vi "DeCoF wait for prompt TCP-socket.vi"(6 "error in (no error)":errorcluster, 7 "time out (ms)":i32=1000, 9 "Connection ID":refnum<k5>) -> (0 "error out":errorcluster, 1 "timed out?":bool, 2 "answer string":string, 3 "Connection ID out":refnum<k5>, 4 "complete answer":string)   [LabVIEW 2013]
doc: "This VI collects the input from the TCP/IP connection until the prompt string is found or the timeout expires.\nThe answer string contains the complete collected string minus the prompt, if found."
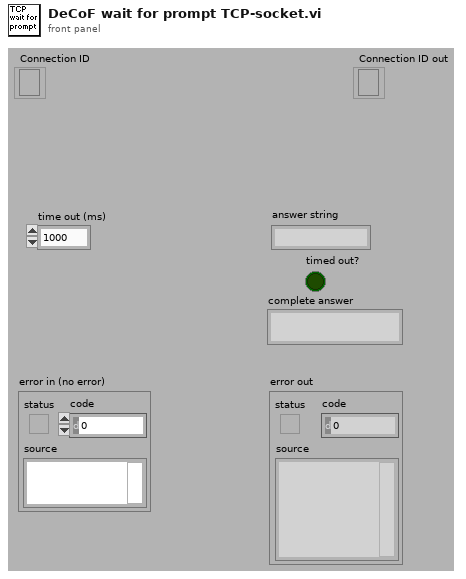
[diagram p1: front panel]
types:
  T1 = enum16{"Standard", "Buffered", "CRLF", "Immediate"}
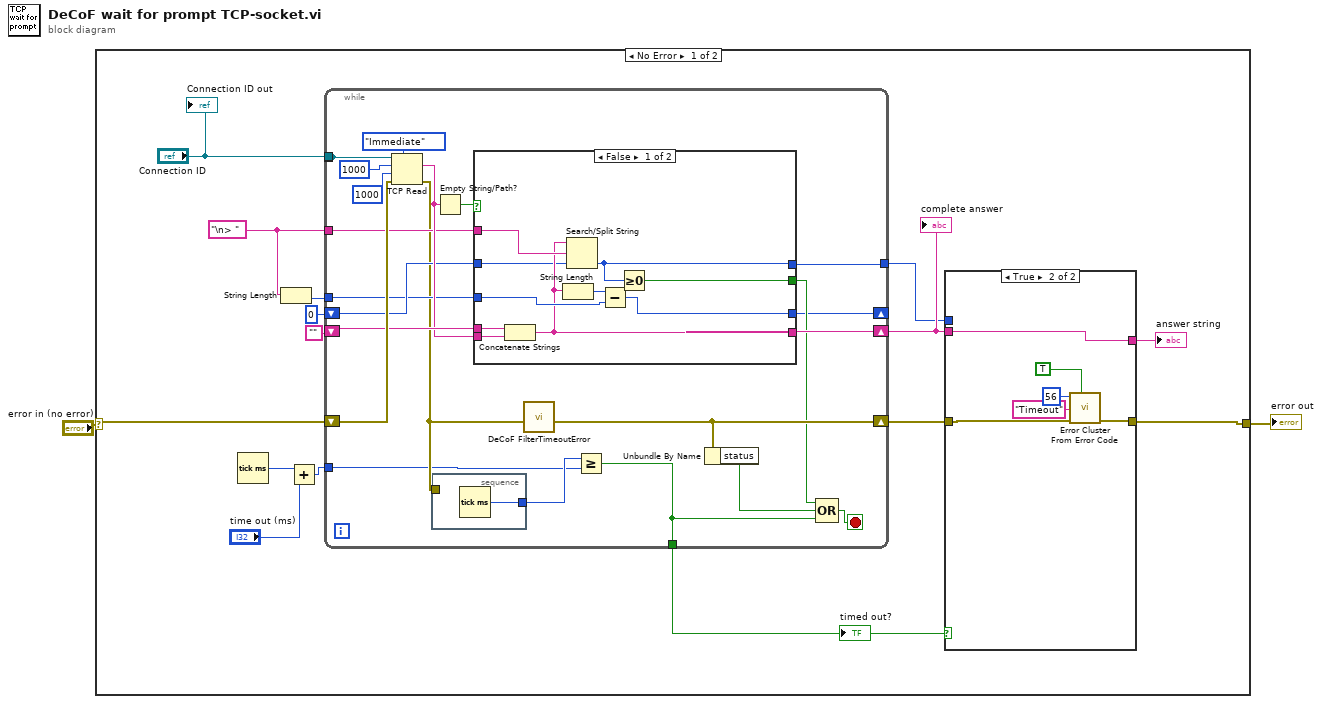
[diagram p0: block diagram]
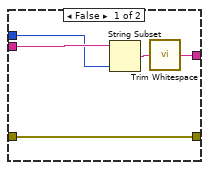
[diagram p2: hidden frame]
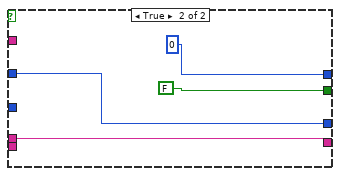
[diagram p3: hidden frame]
diagram:
  n1 = case shown="No Error" "error in (no error)" {
    selector: "error in (no error)" -> [w16 w66]
    tunnel: [w12 w66] -> w1
    frame No Error {
      w9 = "\n> " ("prompt")
      n2 = Tick Count (ms)() -> (millisecond timer value=w7:u32)
      n3 = String Length(string=w9) -> (length=w8:i32)
      n4 = Add(x=w7, y="time out (ms)") -> (x+y=w5:u32)
      n5 = while {
        shift-right: [w41] -> w11
        shift-left: w16 -> [w47]
        tunnel: [w29] -> _
        shift-right: [w35] -> _
        shift-left: 0 -> [w38]
        tunnel: w9 -> [w39]
        shift-right: [w45] -> w14
        shift-left: "" -> [w44]
        tunnel: [w36] -> w10
        tunnel: w8 -> [w34]
        tunnel: w5 -> [w31]
        tunnel: [w30] -> w4
        tunnel: "Connection ID" -> [w29]
        stop <- w50 stop-if-true
        n6 = TCP Read(connection ID=w29, bytes to read=1000, error in (no error)=w47, 7:T1."Immediate" ("mode (standard)"), 9:1000 ("timeout ms (25000)")) -> (data out=w42:string, error out=w33:errorcluster)  [unwired: 1 out]
        n7 = stacked-sequence {
          tunnel: w33 -> [_]
          tunnel: [w51] -> w32
          frame #0 {
            n8 = Tick Count (ms)() -> (millisecond timer value=w51:u32)
          }
        }
        n9 = Empty String/Path?(string/path=w42) -> (empty?=w40:bool)
        n10 = case shown="False" w40 {
          tunnel: [w55 w65] -> w45
          tunnel: w44 -> [w59 w65]
          tunnel: w42 -> [w61 _]
          tunnel: w39 -> [w60 _]
          tunnel: w38 -> [w52 w64]
          tunnel: [w53 FALSE] -> w37
          tunnel: [w54 0 ("offset of match")] -> w36
          tunnel: [w56 w64] -> w35
          tunnel: w34 -> [w57 _]
          frame False {
            n11 = Concatenate Strings(w59, w61) -> (w55:string)
            n12 = String Length(string=w55) -> (length=w58:i32)
            n13 = Search/Split String(string=w55, search string/char (-)=w60, offset (0)=w52) -> (offset of match=w54:i32)  [unwired: 2 out]
            n14 = Subtract(x=w58, y=w57) -> (x-y=w56:i32)
            n15 = Greater Or Equal To 0?(x=w54) -> (x >= 0?=w53:bool)
          }
          frame True {
          }
        }
        n16 = call "DeCoF FilterTimeoutError.vi"("error in (no error)"=w33) -> ("error out"=w41:errorcluster)  [unwired: 5 in, 1 out]
        n17 = Greater Or Equal?(x=w32, y=w31) -> (x >= y?=w30:bool)
        n18 = Unbundle By Name(w41) -> ("status"=w43:bool)
        n19 = Compound Arithmetic op=OR(w37, w43, w30) -> (w50:bool)
      }
      "complete answer" <- w14
      "timed out?" <- w4
      n20 = case shown="True" w4 {
        tunnel: w14 -> [w22 w28]
        tunnel: [w20 w28] -> w13
        tunnel: [w19 w26] -> w12
        tunnel: w11 -> [w19 w27]
        tunnel: w10 -> [w18 _]
        frame False {
          n21 = String Subset(string=w22, length (rest)=w18) -> (substring=w21:string)  [unwired: 1 in]
          n22 = call <vilib>:"Trim Whitespace.vi"("string"=w21) -> ("trimmed string"=w20:string)  [unwired: 1 in]
        }
        frame True {
          n23 = call <vilib>:"Error Cluster From Error Code.vi"("show call chain? (False)"=TRUE, "error in (no error)"=w27, "error message (\"\")"="Timeout" ("error message (\"\")"), "error code (0)"=56) -> ("error out"=w26:errorcluster)  [unwired: 5 in]
        }
      }
      "answer string" <- w13
      "Connection ID out" <- "Connection ID"
    }
    frame Error {
    }
  }
  "error out" <- w1
